vi "Begin.vi"(11 "Image Size":T1=enum."160x120") -> (0 "error out":errorcluster)   [LabVIEW 2012]
doc: "Called before other user functions, this VI is expected to open initial I/O refnums, load in file data, and do all program initialization. Notice that the <B>error out</B> terminal is simply used for data flow. Wiring it to other structures or subVIs ensures that this VI runs first."
uses:
  <vilib>/Rock Robotics/WPI/Camera/WPI_CameraImageSize.ctl
  <vilib>/Rock Robotics/SystemInterfaces/DIO/FPGA_DIOPWMChannel.ctl
  <vilib>/Rock Robotics/WPI/Camera/WPI_CameraWhite Balance Values.ctl
  <vilib>/Rock Robotics/WPI/SafetyOutput/WPI_SafetyOutputConfigMenu.ctl
  <vilib>/Rock Robotics/WPI/DriverStation/WPI_DriverStationRobotMode2.ctl
  <vilib>/Rock Robotics/WPI/Camera/WPI_CameraExposure Values.ctl
  <vilib>/Rock Robotics/WPI/Camera/WPI_CameraFrameRate.ctl
  <vilib>/Rock Robotics/WPI/Joystick/WPI_JoystickDeviceEnum.ctl
  <vilib>/Rock Robotics/SystemInterfaces/AI/FPGA_AIChannel.ctl
  <vilib>/Rock Robotics/WPI/Solenoid/WPI_SolenoidChannel.ctl
  <vilib>/Rock Robotics/SystemInterfaces/DIO/FPGA_DIORelayChannel.ctl
  <vilib>/Rock Robotics/WPI/Relay/WPI_RelayDirection.ctl
  <vilib>/Rock Robotics/SystemInterfaces/DIO/FPGA_DIOChannel.ctl
  <vilib>/Rock Robotics/SystemInterfaces/Typedef/FPGA_TypedefDigitalModule.ctl
  <vilib>/Rock Robotics/WPI/RobotDrive/WPI_RobotDriveOpen2MotorWithTalon.vi
  Robot Global Data.vi
  <vilib>/Rock Robotics/WPI/MotorControl/WPI_MotorControlOpen Victor.vi
  <vilib>/Rock Robotics/WPI/Solenoid/WPI_SolenoidOpenDouble.vi
  <vilib>/Rock Robotics/WPI/MotorControl/WPI_MotorControlOpen Talon.vi
  <vilib>/Rock Robotics/WPI/Counter/WPI_CounterDigitalInputToDigitalSource.vi
panel:
  in  "Image Size 2":T1=enum."160x120"
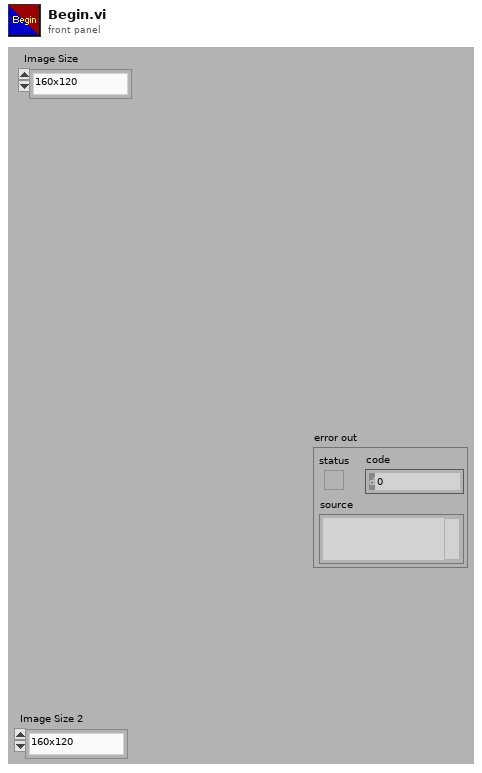
[diagram p1: front panel]
types:
  T1 = typedef "WPI_CameraImageSize.ctl" = enum16{"640x480", "320x240", "160x120"}
  T2 = typedef "WPI_CameraFrameRate.ctl" = u32
  T3 = typedef "WPI_CameraExposure Values.ctl" = enum16{"Auto", "Flicker-free 50 Hz", "Flicker-free 60 Hz", "Hold current"}
  T4 = typedef "WPI_CameraWhite Balance Values.ctl" = enum16{"Auto", "Fixed indoor", "Fixed outdoor 1", "Fixed outdoor 2", "Fixed fluorescent 1", "Fixed fluorescent 2", "Hold current"}
  T5 = typedef "WPI_DriverStationRobotMode2.ctl" = enum16{"Autonomous Disabled", "Autonomous Enabled", "Teleop Disabled", "Teleop Enabled", "Timeout", "Finish", "Test Disabled", "Test Enabled"}
  T6 = typedef "WPI_SafetyOutputConfigMenu.ctl" = enum16{"Enable", "Disable"}
  T7 = typedef "FPGA_DIOPWMChannel.ctl" = enum8{"PWM 1", "PWM 2", "PWM 3", "PWM 4", "PWM 5", "PWM 6", "PWM 7", "PWM 8", "PWM 9", "PWM 10", "Invalid"}
  T8 = typedef "WPI_JoystickDeviceEnum.ctl" = enum16{"USB 1", "USB 2", "USB 3", "USB 4", "Kinect 1", "Kinect 2"}
  T9 = typedef "WPI_JoystickDevRef.ctl" = cluster{"Device":T8}
  T10 = typedef "FPGA_DIOChannel.ctl" = enum8{"DIO 1", "DIO 2", "DIO 3", "DIO 4", "DIO 5", "DIO 6", "DIO 7", "DIO 8", "DIO 9", "DIO 10", "DIO 11", "DIO 12", "DIO 13", "DIO 14", "Invalid"}
  T11 = typedef "FPGA_TypedefDigitalModule.ctl" = enum16{"Digital Module 1", "Digital Module 2"}
  T12 = typedef "WPI_DigitalInputDevRef.ctl" = cluster{"DevStatus":errorcluster, "DIO Channel":T10, "Digital Module":T11}
  T13 = typedef "FPGA_CounterEncoderSourceConvertionLVSourceType.ctl" = cluster{"DevStatus":errorcluster, "AnalogTriggerMode?":bool, "DigitalMode":cluster{"Digital Module":T11, "DIO Channel":T14}, "AnalogTriggerMode":cluster{"AnalogTriggerIndex":T15, "OutputType":T16}}
  T14 = typedef "FPGA_DIODigitalSourceChannel.ctl" = enum8{"DIO 1", "DIO 2", "DIO 3", "DIO 4", "DIO 5", "DIO 6", "DIO 7", "DIO 8", "DIO 9", "DIO 10", "DIO 11", "DIO 12", "DIO 13", "DIO 14", "Disabled"}
  T15 = typedef "FPGA_AnalogTriggerIndex.ctl" = enum8{"Trig 0", "Trig 1", "Trig 2", "Trig 3", "Trig 4", "Trig 5", "Trig 6", "Trig 7", "Invalid"}
  T16 = typedef "FPGA_AnalogTriggerOutType.ctl" = enum16{"InWindow", "TriggerState", "Rising", "Falling"}
  T17 = typedef "WPI_EncoderDevRef.ctl" = cluster{"DevStatus":errorcluster, "EncoderIndex":T18, "CounterIndex":T19, "DistancePerCount":dbl, "Decoding Type":T20}
  T18 = typedef "FPGA_EncoderIdx.ctl" = enum8{"Enc 0", "Enc 1", "Enc 2", "Enc 3", "Invalid"}
  T19 = typedef "FPGA_CounterCtrSystemIndex.ctl" = enum8{"Ctr 0", "Ctr 1", "Ctr 2", "Ctr 3", "Ctr 4", "Ctr 5", "Ctr 6", "Ctr 7", "Invalid"}
  T20 = typedef "WPI_EncoderType.ctl" = enum16{"1x", "2x", "4x"}
  T21 = typedef "WPI_RelayDirection.ctl" = enum16{"Both directions", "Forward only", "Reverse only"}
  T22 = typedef "FPGA_DIORelayChannel.ctl" = enum8{"Relay 1", "Relay 2", "Relay 3", "Relay 4", "Relay 5", "Relay 6", "Relay 7", "Relay 8", "Invalid"}
  T23 = typedef "WPI_RelayDevRef.ctl" = cluster{"DevStatus":errorcluster, "Relay Channel":T22, "Digital Module":T11, "Relay Direction":T21}
  T24 = typedef "WPI_ServoDeviceRef.ctl" = cluster{"DeviceStatus":errorcluster, "Digital Module":T11, "PWM Channel":T7, "DeadBand":T25}
  T25 = typedef "WPI_PWMDeadband.ctl" = cluster{"Name":string, "maxPositivePwm":i32, "minPositivePwm":i32, "centerPwm":i32, "maxNegativePwm":i32, "minNegativePwm":i32, "angularRange":u16}
  T26 = typedef "WPI_SolenoidChannel.ctl" = enum8{"Solenoid 1", "Solenoid 2", "Solenoid 3", "Solenoid 4", "Solenoid 5", "Solenoid 6", "Solenoid 7", "Solenoid 8", "Invalid"}
  T27 = typedef "WPI_MotorControlDeviceRef.ctl" = cluster{"DeviceStatus":errorcluster, "Type":enum16{"PWM", "CAN"}, "PWM":cluster{"Digital Module":T11, "PWM Channel":T7, "DeadBand":T25}, "CAN":cluster{"Device Number":u8, "Control Mode":T28, "Semaphore":T29, "Max Vout":dbl}, "Invert":bool, "TransformRef":T30, "InvTransformRef":T30}
  T28 = typedef "WPI_CANJaguar_ControlMode.ctl" = enum8{"Percent VBus", "Current", "Speed", "Position", "Voltage"}
  T29 = typedef "Semaphore RefNum" = refnum<k1>
  T30 = typedef "WPI_PWMTransform_ConPane.ctl" = refnum<vi>
  T31 = typedef "WPI_SolenoidDevRef.ctl" = cluster{"DevStatus":errorcluster, "Solenoid Module":T32, "Forward Solenoid Channel":T26, "Reverse Solenoid Channel":T26}
  T32 = typedef "FPGA_TypedefSolenoidModule.ctl" = enum16{"Solenoid Module 1", "Solenoid Module 2"}
  T33 = typedef "FPGA_AIChannel.ctl" = enum8{"AI 1", "AI 2", "AI 3", "AI 4", "AI 5", "AI 6", "AI 7", "AI 8", "Invalid"}
  T34 = typedef "WPI_AnalogChannelDevRef.ctl" = cluster{"DevStatus":errorcluster, "Analog Module":T35, "Analog Channel":T33}
  T35 = typedef "FPGA_TypedefAnalogModule.ctl" = enum16{"Analog Module 1", "Analog Module 2"}
  T36 = typedef "WPI_CameraDevRef.ctl" = cluster{"Camera Address":string, "CameraStatus":errorcluster, "Acquire Image Notifier":refnum<notifier>}
  T37 = typedef "WPI_RobotDriveDevRef.ctl" = cluster{"DevStatus":errorcluster, "Motors[]":T27[], "Square Inputs":bool, "Max Output":dbl, "Isochronous":bool}
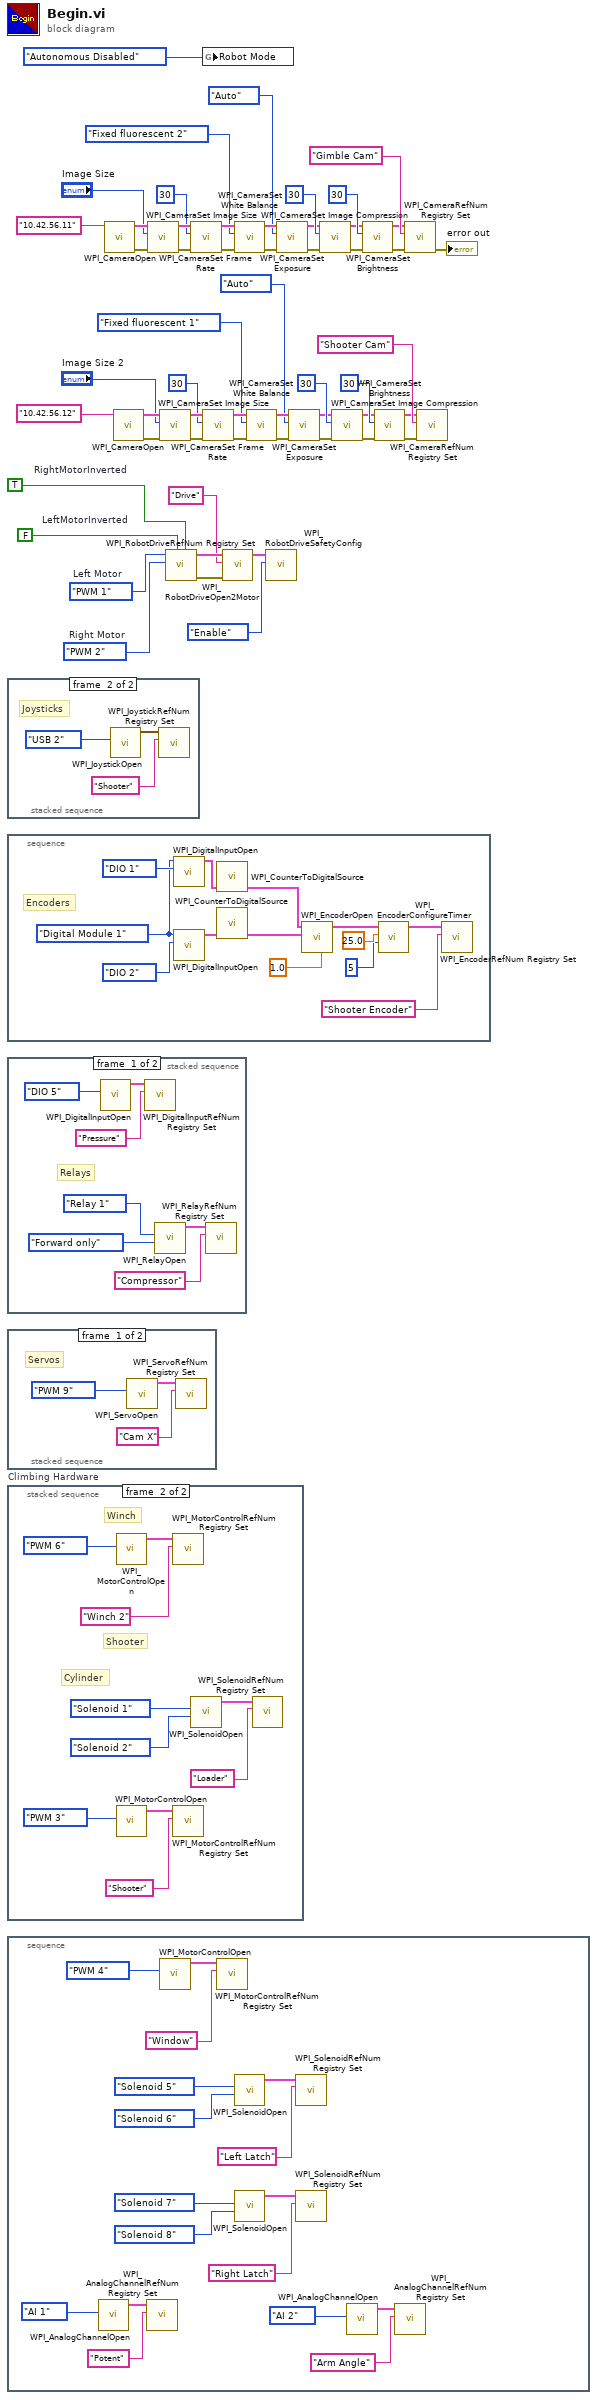
[diagram p0: block diagram]
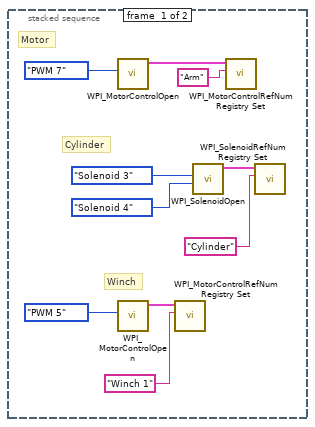
[diagram p2: hidden frame]
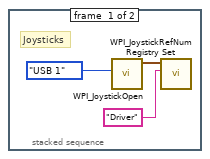
[diagram p3: hidden frame]
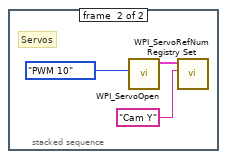
[diagram p4: hidden frame]
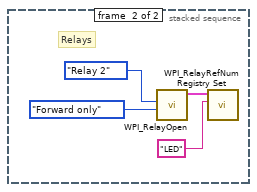
[diagram p5: hidden frame]
diagram:
  w31 = FPGA_DIOPWMChannel."PWM 2"  # Right Motor
  w32 = FPGA_DIOPWMChannel."PWM 1"  # Left Motor
  w54 = FALSE  # LeftMotorInverted
  w55 = TRUE  # RightMotorInverted
  n1 = stacked-sequence {
    frame #0 {
      # "Joysticks"
      n2 = call <vilib>:"WPI_JoystickOpen.vi"("JoystickDevice"=WPI_JoystickDeviceEnum."USB 1") -> ("JoystickDevRef"=w57:T9)  [unwired: 10 in]
      n3 = call <vilib>:"WPI_JoystickRefNum Registry Set.vi"("refnum name"="Driver", "JoystickDevRef"=w57) -> ()  [unwired: 8 in, 2 out]
    }
    frame #1 {
      # "Joysticks"
      n4 = call <vilib>:"WPI_JoystickOpen.vi"("JoystickDevice"=WPI_JoystickDeviceEnum."USB 2") -> ("JoystickDevRef"=w60:T9)  [unwired: 10 in]
      n5 = call <vilib>:"WPI_JoystickRefNum Registry Set.vi"("refnum name"="Shooter", "JoystickDevRef"=w60) -> ()  [unwired: 8 in, 2 out]
    }
  }
  n6 = stacked-sequence {
    frame #0 {
      w68 = FPGA_TypedefDigitalModule."Digital Module 1" ("Digital Module (Module 1)")
      # "Encoders"
      n7 = call <vilib>:"WPI_DigitalInputOpen.vi"("DIO Channel"=FPGA_DIOChannel."DIO 1", "Digital Module (Module 1)"=w68) -> ("DigitalInputDevRef"=w74:T12)  [unwired: 8 in, 1 out]
      n8 = call <vilib>:"WPI_DigitalInputOpen.vi"("DIO Channel"=FPGA_DIOChannel."DIO 2", "Digital Module (Module 1)"=w68) -> ("DigitalInputDevRef"=w70:T12)  [unwired: 8 in, 1 out]
      n9 = call-poly <vilib>:"WPI_CounterToDigitalSource.vi"("DigitalInputDevRef"=w74) -> ("Digital Source"=w73:T13)  [unwired: 6 in]
      n10 = call-poly <vilib>:"WPI_CounterToDigitalSource.vi"("DigitalInputDevRef"=w70) -> ("Digital Source"=w69:T13)  [unwired: 6 in]
      n11 = call <vilib>:"WPI_EncoderOpen.vi"("DistancePerCount"=1.0, "BSource"=w69, "ASource"=w73) -> ("EncoderDevRef"=w66:T17)  [unwired: 7 in, 1 out]
      n12 = call <vilib>:"WPI_EncoderConfigureTimer.vi"("Number Samples to Average"=u8 5, "Minimum Rate"=25.0, "EncoderDevRef"=w66) -> ("EncoderDevRef"=w65:T17)  [unwired: 7 in, 1 out]
      n13 = call <vilib>:"WPI_EncoderRefNum Registry Set.vi"("refnum name"="Shooter Encoder", "EncoderDevRef"=w65) -> ()  [unwired: 8 in, 2 out]
    }
  }
  n14 = stacked-sequence {
    frame #0 {
      # "Relays"
      n15 = call <vilib>:"WPI_DigitalInputOpen.vi"("DIO Channel"=FPGA_DIOChannel."DIO 5") -> ("DigitalInputDevRef"=w76:T12)  [unwired: 9 in, 1 out]
      n16 = call <vilib>:"WPI_DigitalInputRefNum Registry Set.vi"("refnum name"="Pressure", "DigitalInputDevRef"=w76) -> ()  [unwired: 8 in, 2 out]
      n17 = call <vilib>:"WPI_RelayOpen.vi"("Relay Direction"=WPI_RelayDirection."Forward only", "Relay Channel"=FPGA_DIORelayChannel."Relay 1") -> ("RelayDevRef"=w81:T23)  [unwired: 8 in, 1 out]
      n18 = call <vilib>:"WPI_RelayRefNum Registry Set.vi"("refnum name"="Compressor", "RelayDevRef"=w81) -> ()  [unwired: 8 in, 2 out]
    }
    frame #1 {
      # "Relays"
      n19 = call <vilib>:"WPI_RelayOpen.vi"("Relay Direction"=WPI_RelayDirection."Forward only", "Relay Channel"=FPGA_DIORelayChannel."Relay 2") -> ("RelayDevRef"=w85:T23)  [unwired: 8 in, 1 out]
      n20 = call <vilib>:"WPI_RelayRefNum Registry Set.vi"("refnum name"="LED", "RelayDevRef"=w85) -> ()  [unwired: 8 in, 2 out]
    }
  }
  n21 = stacked-sequence {
    frame #0 {
      # "Servos"
      n22 = call <vilib>:"WPI_ServoOpen.vi"("PWM Channel"=FPGA_DIOPWMChannel."PWM 9") -> ("ServoDeviceRef"=w88:T24)  [unwired: 9 in, 1 out]
      n23 = call <vilib>:"WPI_ServoRefNum Registry Set.vi"("refnum name"="Cam X", "ServoDeviceRef"=w88) -> ()  [unwired: 8 in, 2 out]
    }
    frame #1 {
      # "Servos"
      n24 = call <vilib>:"WPI_ServoOpen.vi"("PWM Channel"=FPGA_DIOPWMChannel."PWM 10") -> ("ServoDeviceRef"=w89:T24)  [unwired: 9 in, 1 out]
      n25 = call <vilib>:"WPI_ServoRefNum Registry Set.vi"("refnum name"="Cam Y", "ServoDeviceRef"=w89) -> ()  [unwired: 8 in, 2 out]
    }
  }
  n26 = stacked-sequence "Climbing Hardware" {
    frame #0 {
      # "Motor"
      # "Cylinder"
      # "Winch"
      n27 = call-poly <vilib>:"WPI_MotorControlOpen.vi"("PWM Channel"=FPGA_DIOPWMChannel."PWM 7") -> ("MotorControlDeviceRef"=w93:T27)  [unwired: 9 in, 1 out]
      n28 = call-poly <vilib>:"WPI_MotorControlOpen.vi"("PWM Channel"=FPGA_DIOPWMChannel."PWM 5") -> ("MotorControlDeviceRef"=w100:T27)  [unwired: 9 in, 1 out]
      n29 = call <vilib>:"WPI_MotorControlRefNum Registry Set.vi"("refnum name"="Winch 1", "MotorControlDevRef"=w100) -> ()  [unwired: 8 in, 2 out]
      n30 = call-poly <vilib>:"WPI_SolenoidOpen.vi"("Reverse Solenoid Channel"=WPI_SolenoidChannel."Solenoid 4", "Forward Solenoid Channel"=WPI_SolenoidChannel."Solenoid 3") -> ("SolenoidDevRef"=w95:T31)  [unwired: 8 in, 1 out]
      n31 = call <vilib>:"WPI_MotorControlRefNum Registry Set.vi"("refnum name"="Arm", "MotorControlDevRef"=w93) -> ()  [unwired: 8 in, 2 out]
      n32 = call <vilib>:"WPI_SolenoidRefNum Registry Set.vi"("refnum name"="Cylinder", "SolenoidDevRef"=w95) -> ()  [unwired: 8 in, 2 out]
    }
    frame #1 {
      # "Cylinder"
      # "Shooter"
      # "Winch"
      n33 = call-poly <vilib>:"WPI_MotorControlOpen.vi"("PWM Channel"=FPGA_DIOPWMChannel."PWM 6") -> ("MotorControlDeviceRef"=w110:T27)  [unwired: 9 in, 1 out]
      n34 = call-poly <vilib>:"WPI_MotorControlOpen.vi"("PWM Channel"=FPGA_DIOPWMChannel."PWM 3") -> ("MotorControlDeviceRef"=w107:T27)  [unwired: 9 in, 1 out]
      n35 = call <vilib>:"WPI_MotorControlRefNum Registry Set.vi"("refnum name"="Winch 2", "MotorControlDevRef"=w110) -> ()  [unwired: 8 in, 2 out]
      n36 = call <vilib>:"WPI_MotorControlRefNum Registry Set.vi"("refnum name"="Shooter", "MotorControlDevRef"=w107) -> ()  [unwired: 8 in, 2 out]
      n37 = call-poly <vilib>:"WPI_SolenoidOpen.vi"("Reverse Solenoid Channel"=WPI_SolenoidChannel."Solenoid 2", "Forward Solenoid Channel"=WPI_SolenoidChannel."Solenoid 1") -> ("SolenoidDevRef"=w103:T31)  [unwired: 8 in, 1 out]
      n38 = call <vilib>:"WPI_SolenoidRefNum Registry Set.vi"("refnum name"="Loader", "SolenoidDevRef"=w103) -> ()  [unwired: 8 in, 2 out]
    }
  }
  n39 = stacked-sequence {
    frame #0 {
      n40 = call <vilib>:"WPI_AnalogChannelOpen.vi"("Analog Channel"=FPGA_AIChannel."AI 1") -> ("AIDeviceRef"=w126:T34)  [unwired: 9 in, 1 out]
      n41 = call <vilib>:"WPI_AnalogChannelRefNum Registry Set.vi"("refnum name"="Potent", "AIDeviceRef"=w126) -> ()  [unwired: 8 in, 2 out]
      n42 = call-poly <vilib>:"WPI_MotorControlOpen.vi"("PWM Channel"=FPGA_DIOPWMChannel."PWM 4") -> ("MotorControlDeviceRef"=w125:T27)  [unwired: 9 in, 1 out]
      n43 = call <vilib>:"WPI_MotorControlRefNum Registry Set.vi"("refnum name"="Window", "MotorControlDevRef"=w125) -> ()  [unwired: 8 in, 2 out]
      n44 = call-poly <vilib>:"WPI_SolenoidOpen.vi"("Reverse Solenoid Channel"=WPI_SolenoidChannel."Solenoid 6", "Forward Solenoid Channel"=WPI_SolenoidChannel."Solenoid 5") -> ("SolenoidDevRef"=w122:T31)  [unwired: 8 in, 1 out]
      n45 = call-poly <vilib>:"WPI_SolenoidOpen.vi"("Reverse Solenoid Channel"=WPI_SolenoidChannel."Solenoid 8", "Forward Solenoid Channel"=WPI_SolenoidChannel."Solenoid 7") -> ("SolenoidDevRef"=w115:T31)  [unwired: 8 in, 1 out]
      n46 = call <vilib>:"WPI_SolenoidRefNum Registry Set.vi"("refnum name"="Left Latch", "SolenoidDevRef"=w122) -> ()  [unwired: 8 in, 2 out]
      n47 = call <vilib>:"WPI_SolenoidRefNum Registry Set.vi"("refnum name"="Right Latch", "SolenoidDevRef"=w115) -> ()  [unwired: 8 in, 2 out]
      n48 = call <vilib>:"WPI_AnalogChannelOpen.vi"("Analog Channel"=FPGA_AIChannel."AI 2") -> ("AIDeviceRef"=w112:T34)  [unwired: 9 in, 1 out]
      n49 = call <vilib>:"WPI_AnalogChannelRefNum Registry Set.vi"("refnum name"="Arm Angle", "AIDeviceRef"=w112) -> ()  [unwired: 8 in, 2 out]
    }
  }
  n50 = call <vilib>:"WPI_CameraOpen.vi"("Camera Address"="10.42.56.11") -> ("error out"=w41:errorcluster, "CameraDevRef"=w42:T36)  [unwired: 1 in, 8 out]
  n51 = call <vilib>:"WPI_CameraOpen.vi"("Camera Address"="10.42.56.12") -> ("error out"=w14:errorcluster, "CameraDevRef"=w15:T36)  [unwired: 1 in, 8 out]
  n52 = call <vilib>:"WPI_CameraSet Image Size.vi"("error in (no error)"=w41, "Image Size"="Image Size", "CameraDevRef"=w42) -> ("error out"=w40:errorcluster, "CameraDevRef Out"=w43:T36)  [unwired: 7 out]
  n53 = call <vilib>:"WPI_CameraSet Image Size.vi"("error in (no error)"=w14, "Image Size"="Image Size 2", "CameraDevRef"=w15) -> ("error out"=w13:errorcluster, "CameraDevRef Out"=w16:T36)  [unwired: 7 out]
  n54 = call-poly <vilib>:"WPI_RobotDriveOpen2Motor.vi"("Right Motor Inverted"=w55, "Left Motor Inverted"=w54, "Right Motor"=w31, "Left Motor"=w32) -> ("error out"=w50:errorcluster, "RobotDriveDevRef"=w52:T37)  [unwired: 1 in, 5 out]
  n55 = call <vilib>:"WPI_CameraSet Frame Rate.vi"("error in (no error)"=w40, "Frame Rate (fps)"=T2 30, "CameraDevRef"=w43) -> ("error out"=w39:errorcluster, "CameraDevRef Out"=w45:T36)  [unwired: 7 out]
  n56 = global write "Robot Global Data.vi" "Robot Mode"(WPI_DriverStationRobotMode2."Autonomous Disabled" ("Robot Mode")) -> ()
  n57 = call <vilib>:"WPI_CameraSet Frame Rate.vi"("error in (no error)"=w13, "Frame Rate (fps)"=T2 30, "CameraDevRef"=w16) -> ("error out"=w12:errorcluster, "CameraDevRef Out"=w18:T36)  [unwired: 7 out]
  n58 = call <vilib>:"WPI_RobotDriveRefNum Registry Set.vi"("error in (no error)"=w50, "refnum name"="Drive", "RobotDriveDevRef"=w52) -> ("RobotDriveDevRef"=w27:T37)  [unwired: 8 out]
  n59 = call <vilib>:"WPI_CameraSet White Balance.vi"("error in (no error)"=w39, "White Balance"=WPI_CameraWhite_Balance_Values."Fixed fluorescent 2", "CameraDevRef"=w45) -> ("error out"=w38:errorcluster, "CameraDevRef Out"=w44:T36)  [unwired: 7 out]
  n60 = call <vilib>:"WPI_CameraSet White Balance.vi"("error in (no error)"=w12, "White Balance"=WPI_CameraWhite_Balance_Values."Fixed fluorescent 1", "CameraDevRef"=w18) -> ("error out"=w11:errorcluster, "CameraDevRef Out"=w17:T36)  [unwired: 7 out]
  n61 = call <vilib>:"WPI_RobotDriveSafetyConfig.vi"("mode"=WPI_SafetyOutputConfigMenu."Enable", "RobotDriveDevRef"=w27) -> ()  [unwired: 8 in, 2 out]
  n62 = call <vilib>:"WPI_CameraSet Exposure.vi"("error in (no error)"=w38, "Exposure"=WPI_CameraExposure_Values."Auto", "CameraDevRef"=w44) -> ("error out"=w37:errorcluster, "CameraDevRef Out"=w47:T36)  [unwired: 7 out]
  n63 = call <vilib>:"WPI_CameraSet Exposure.vi"("error in (no error)"=w11, "Exposure"=WPI_CameraExposure_Values."Auto", "CameraDevRef"=w17) -> ("error out"=w10:errorcluster, "CameraDevRef Out"=w20:T36)  [unwired: 7 out]
  n64 = call <vilib>:"WPI_CameraSet Image Compression.vi"("error in (no error)"=w37, "Compression"=30, "CameraDevRef"=w47) -> ("error out"=w36:errorcluster, "CameraDevRef Out"=w46:T36)  [unwired: 7 out]
  n65 = call <vilib>:"WPI_CameraSet Image Compression.vi"("error in (no error)"=w10, "Compression"=30, "CameraDevRef"=w20) -> ("error out"=w9:errorcluster, "CameraDevRef Out"=w19:T36)  [unwired: 7 out]
  n66 = call <vilib>:"WPI_CameraSet Brightness.vi"("error in (no error)"=w36, "Brightness"=30, "CameraDevRef"=w46) -> ("error out"=w34:errorcluster, "CameraDevRef Out"=w35:T36)  [unwired: 7 out]
  n67 = call <vilib>:"WPI_CameraSet Brightness.vi"("error in (no error)"=w9, "Brightness"=30, "CameraDevRef"=w19) -> ("error out"=w7:errorcluster, "CameraDevRef Out"=w8:T36)  [unwired: 7 out]
  n68 = call <vilib>:"WPI_CameraRefNum Registry Set.vi"("error in (no error)"=w34, "refnum name"="Gimble Cam", "CameraDevRef"=w35) -> ("error out"=→"error out":errorcluster)  [unwired: 8 out]
  n69 = call <vilib>:"WPI_CameraRefNum Registry Set.vi"("error in (no error)"=w7, "refnum name"="Shooter Cam", "CameraDevRef"=w8) -> ()  [unwired: 9 out]
